vi "p02 Integer Math (Host).vi"() -> ()   [LabVIEW 2025]
uses:
  <vilib>/rvi/interface/nirviOpenFPGA/nirviOpenFPGA.xnode
  <vilib>/rvi/interface/nirviReadWriteControl/nirviReadWriteControl.xnode
  <vilib>/rvi/interface/nirviCloseFPGA/nirviCloseFPGA.xnode
  <vilib>/rvi/interface/RandomDataEmulation/nirviRandomDataOpen.vi
  <vilib>/rvi/interface/common/niFpgaCacheSessionInfoDynamic.vi
  <vilib>/FPGAPlugInAG/Dynamic/niLvFpga_Close_Dynamic.vi
  NiFpgaLv.dll
  <vilib>/Utility/error.llb/Error Cluster From Error Code.vi
  <vilib>/rvi/interface/Simulation/niFpgaSimulationCallBeginRW.vi
  <vilib>/rvi/errors/niLvFpgaAdjustHostInterfaceError.vi
panel:
  out "Scaled":dbl(graph)
  out "Connector1/AI0":dbl(graph)
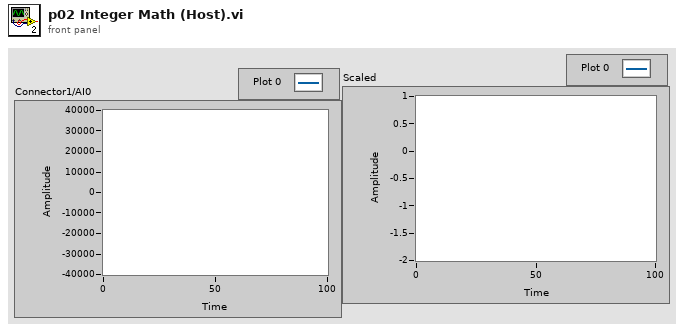
[diagram p1: front panel]
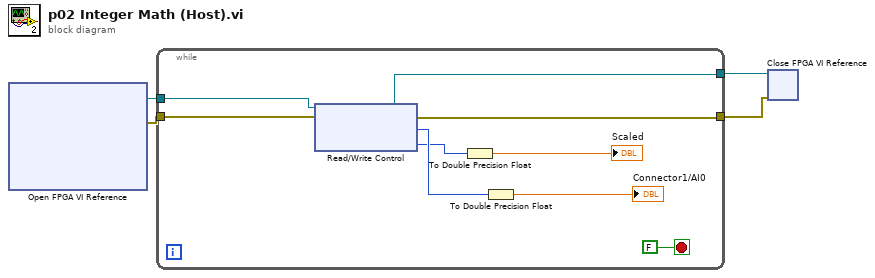
[diagram p0: block diagram]
diagram:
  n1 = xnode "Open FPGA VI Reference"() -> ("FPGA VI Reference Out"=w4:refnum<k20>, "error out"=w2:errorcluster)  [unwired: 2 in]
  n2 = while {
    tunnel: w4 -> [w13]
    tunnel: [w12] -> w3
    tunnel: w2 -> [w11]
    tunnel: [w10] -> w1
    stop <- FALSE stop-if-true
    n3 = xnode "Read/Write Control"("FPGA VI Reference In"=w13, "error in"=w11) -> ("FPGA VI Reference Out"=w12:refnum<k20>, "error out"=w10:errorcluster, "Connector1/AI0"=w9:i16, "Scaled"=w5:i16)
    n4 = To Double Precision Float(number=w5) -> (double precision float=→"Scaled":dbl)
    n5 = To Double Precision Float(number=w9) -> (double precision float=→"Connector1/AI0":dbl)
  }
  n6 = xnode "Close FPGA VI Reference"("FPGA VI Reference In"=w3, "error in"=w1) -> ()  [unwired: 1 out]
